vi "Set Discharge Switch.vi"(0 "reference in":refnum<class "Battery.lvclass">, 2 "Discharge Switch":bool, 5 "Error In":errorcluster) -> (14 "reference out":refnum<class "Battery.lvclass">, 19 "Error Out":errorcluster)   [LabVIEW 2023, in "Battery.lvclass"]
uses:
  Battery.lvclass
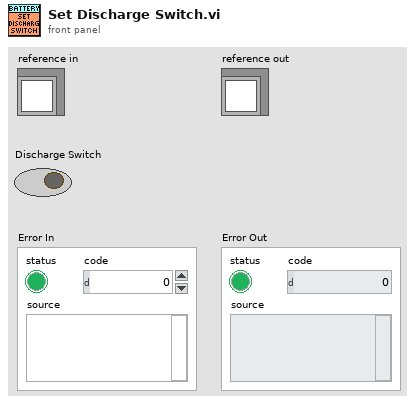
[diagram p1: front panel]
types:
  T1 = enum16{"Disconnected", "Charging", "Discharging"}
  T2 = typedef "Battery.lvclass/ObjectAttributes.ctl" = cluster{"Mode":enum16{"Disconnected", "Charging", "Discharging"}, "Discharge Switch":bool, "Allow Charging":bool, "Cell Voltage (V)":dbl, "Cell Current (A)":dbl, "SoC (%)":dbl, "Nominal Voltage (V)":dbl, "Model Index":i32, "Charge Model":cluster{"Voltage (V)":dbl[], "Current (A)":dbl[], "SoC (%)":dbl[]}, "Discharge Model":cluster{"Voltage (V)":dbl[], "Current (A)":dbl[], "SoC (%)":dbl[]}, "Simulation Error":errorcluster}
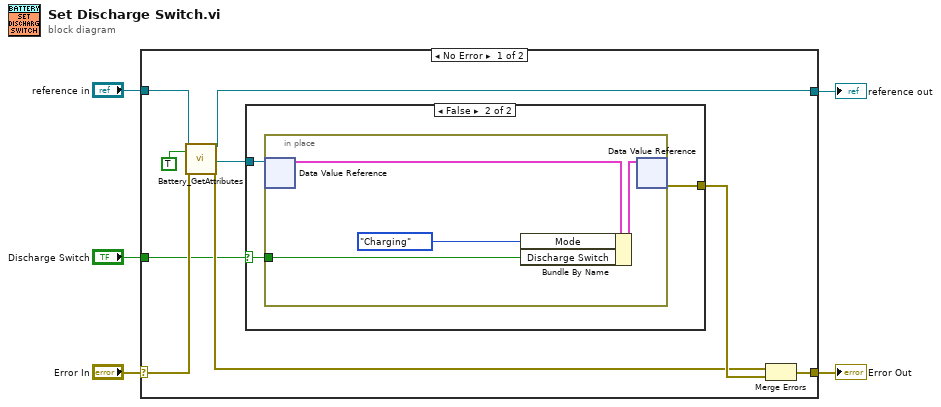
[diagram p0: block diagram]
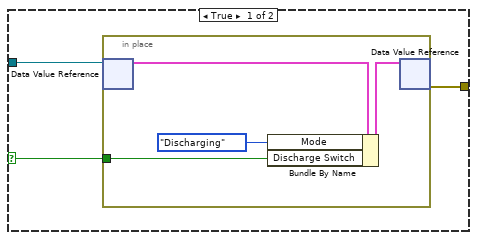
[diagram p2: hidden frame]
diagram:
  n1 = case shown="No Error" "Error In" {
    selector: "Error In" -> [w14 w30]
    tunnel: [w11 w30] -> w4
    tunnel: [w9 w29] -> w2
    tunnel: "reference in" -> [w10 w29]
    tunnel: "Discharge Switch" -> [w6 _]
    frame No Error {
      n2 = call "Battery_GetAttributes.vi"("reference in"=w10, "OnlyGetDvrReference(False)"=TRUE, "Error In"=w14) -> ("reference out"=w9:refnum<class "Battery.lvclass">, "DataRef"=w7:refnum<data-value>, "Error Out"=w12:errorcluster)  [unwired: 13 in, 1 out]
      n3 = case shown="False" w6 {
        selector: w6 -> [w15 w22]
        tunnel: [w17 w24] -> w13
        tunnel: w7 -> [w16 w23]
        frame True {
          n4 = in-place {
            in-place-border: w15 -> [w19]
            n5 = in-place-dvr #1(w16) -> (w21:T2)  [unwired: 1 out]
            n6 = Bundle By Name(cluster=w21, "Mode"=T1."Discharging", "Discharge Switch"=w19) -> (w20:T2)
            n7 = in-place-dvr #1(w20) -> (w17:errorcluster)  [unwired: 1 out]
          }
        }
        frame False {
          n8 = in-place {
            in-place-border: w22 -> [w27]
            n9 = in-place-dvr #2(w23) -> (w26:T2)  [unwired: 1 out]
            n10 = Bundle By Name(cluster=w26, "Mode"=T1."Charging" ("t"), "Discharge Switch"=w27) -> (w28:T2)
            n11 = in-place-dvr #2(w28) -> (w24:errorcluster)  [unwired: 1 out]
          }
        }
      }
      n12 = Merge Errors(w12, w13) -> (w11:errorcluster)
    }
    frame Error {
    }
  }
  "Error Out" <- w4
  "reference out" <- w2
